vi "Init_CtlLookupClass.vi"(8 "error in (no error)":errorcluster) -> (0 "error out":errorcluster, 3 "CtlLookup":T1)   [LabVIEW 2020, in "CtlReferences.lvlib" / "CtlReferences.lvclass"]
uses:
  CtlReferences.lvclass
  TypeDefs/CtlLookup.ctl
  CtlReferences.lvclass/CtlReferences.ctl
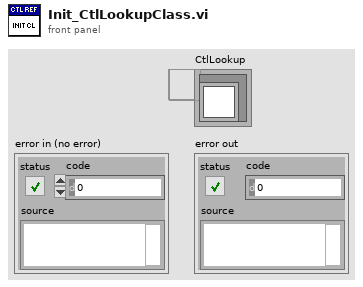
[diagram p1: front panel]
types:
  T1 = typedef "CtlReferences.lvlib/CtlReferences.lvclass/CtlLookup.ctl" = refnum<data-value>
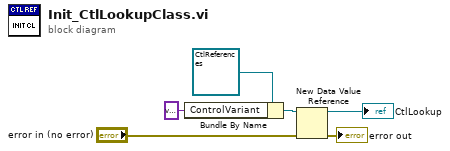
[diagram p0: block diagram]
diagram:
  n1 = Bundle By Name(cluster=refnum<class "CtlReferences.lvclass"> refnum ("CtlReferences.lvclass"), "ControlVariant"=variant) -> (w2:refnum<class "CtlReferences.lvclass">)
  n2 = New Data Value Reference(data value=w2, error in="error in (no error)") -> (data value reference=→"CtlLookup":refnum<data-value>, error out=→"error out":errorcluster)
